vi "Set Emtype SN.vi"(11 "数值":dbl) -> (2 "OUT STR":string, 3 "NA SN":string[](array[string]))   [LabVIEW 2018]
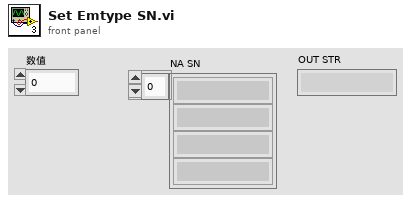
[diagram p1: front panel]
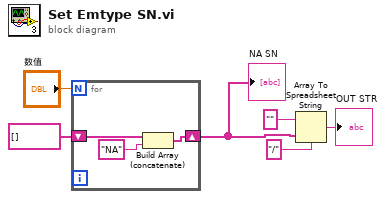
[diagram p0: block diagram]
diagram:
  n1 = for {
    N: "数值" -> [_]
    shift-right: [w8] -> w2
    shift-left: string[] [] -> [w9]
    n2 = Build Array (concatenate)(w9, "NA") -> (w8:string[])
  }
  "NA SN" <- w2
  n3 = Array To Spreadsheet String(delimiter (Tab)="/" ("分隔符(Tab)"), array=w2, 3:"" ("格式字符串")) -> (spreadsheet string=→"OUT STR":string)
